vi "Check All Bcklg Reg New.vi"(7 "TimingEngine":T1, 8 "error in (no error)":errorcluster, 11 "FP Controls in":refnum<class "FP Controls.lvclass">) -> (0 "error out":errorcluster, 1 "Max Bcklg":dbl, 2 "Update FP?":bool, 3 "FP Controls out":refnum<class "FP Controls.lvclass">)   [LabVIEW 2018, in "Configuration Grandmaster.lvlib" / "FP Controls.lvclass"]
uses:
  FP Controls.lvclass
  Common/Controls/TE_Designator.ctl
  FP Controls.lvclass/FP Controls.ctl
  Common/Controls/DAQ Diagnostics.ctl
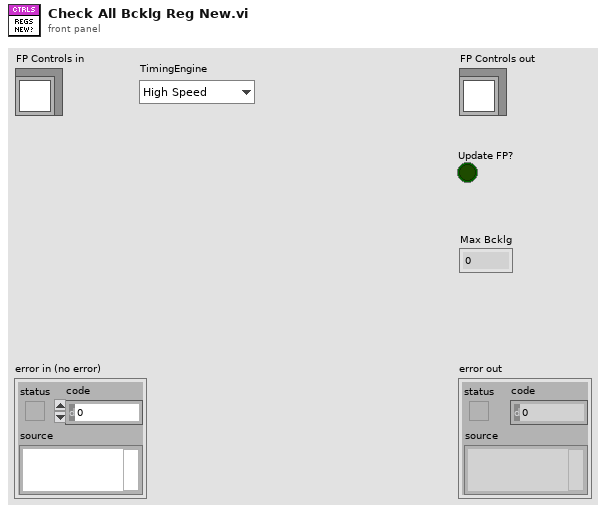
[diagram p1: front panel]
types:
  T1 = typedef "TE_Designator.ctl" = enum16{"High Speed", "Low Speed"}
  T2 = typedef "DAQ Diagnostics.ctl" = cluster{"New":bool, "LoopRate (ms)":u32, "Bff Bcklg":dbl}
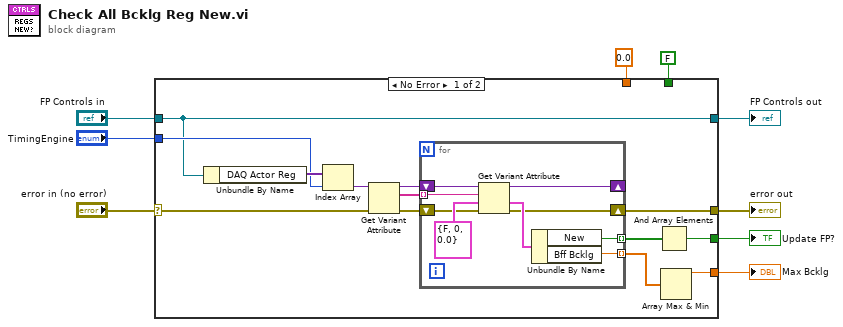
[diagram p0: block diagram]
diagram:
  n1 = case shown="No Error" "error in (no error)" {
    selector: "error in (no error)" -> [w22 w35]
    tunnel: [w21 w35] -> w8
    tunnel: [w13 w34] -> w6
    tunnel: "FP Controls in" -> [w13 w34]
    tunnel: "TimingEngine" -> [w15 _]
    tunnel: [w11 w33] -> w4
    tunnel: [w10 w32] -> w3
    tunnel: FALSE -> [_ w33]
    tunnel: 0.0 -> [_ w32]
    frame No Error {
      n2 = Unbundle By Name(w13) -> ("DAQ Actor Reg"=w20:variant[])
      n3 = Index Array(array=w20, index=w15) -> (element=w16:variant)
      n4 = Get Variant Attribute(Variant=w16, error in=w22) -> (duplicate Variant=w18:variant, names=w19:string[], error out=w17:errorcluster)  [unwired: 2 in, 1 out]
      n5 = for {
        tunnel: w19 -> [w30] mode=indexing
        shift-right: [w24] -> _
        shift-left: w18 -> [w31]
        shift-right: [w23] -> w21
        shift-left: w17 -> [w28]
        tunnel: [w26] -> w14 mode=indexing
        tunnel: [w25] -> w12 mode=indexing
        n6 = Get Variant Attribute(Variant=w31, name=w30, default value (empty Variant)=T2 {"New"=FALSE, "LoopRate (ms)"=0, "Bff Bcklg"=0.0} ("DAQ Diag"), error in=w28) -> (duplicate Variant=w24:variant, value=w27:T2, error out=w23:errorcluster)  [unwired: 1 out]
        n7 = Unbundle By Name(w27) -> ("New"=w26:bool, "Bff Bcklg"=w25:dbl)
      }
      n8 = And Array Elements(Boolean array=w14) -> (logical AND=w11:bool)
      n9 = Array Max & Min(array=w12) -> (max value=w10:dbl)  [unwired: 3 out]
    }
    frame Error {
    }
  }
  "error out" <- w8
  "FP Controls out" <- w6
  "Update FP?" <- w4
  "Max Bcklg" <- w3
